vi "test Unpause timer reports the correct time.vi"(8 "error in (no error)":errorcluster, 11 "TestCase in":refnum<class "Test Unpause Timer.lvclass">) -> (0 "error out":errorcluster, 3 "TestCase out":refnum<class "Test Unpause Timer.lvclass">)   [LabVIEW 2018, in "Test Unpause Timer.lvclass"]
uses:
  Test Unpause Timer.lvclass
  Test Unpause Timer.lvclass/Test Unpause Timer.ctl
  <vilib>/addons/_JKI Toolkits/VI Tester/TestCase.llb/TestCase.lvclass
  C:/Program Files (x86)/National Instruments/LabVIEW 2018/vi.lib/addons/_JKI Toolkits/VI Tester/TestCase.llb/TestCase.lvclass
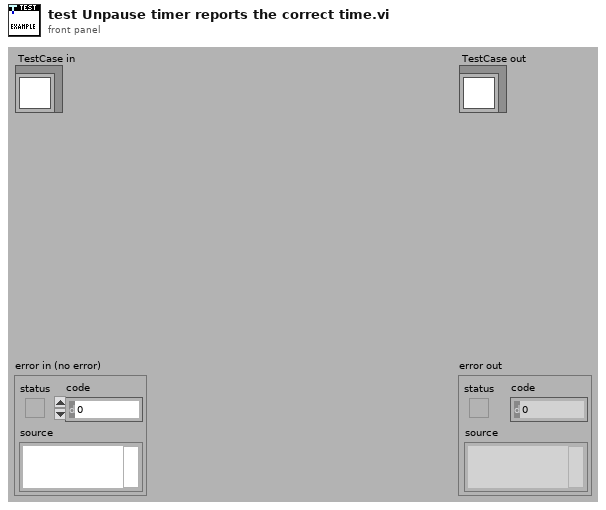
[diagram p1: front panel]
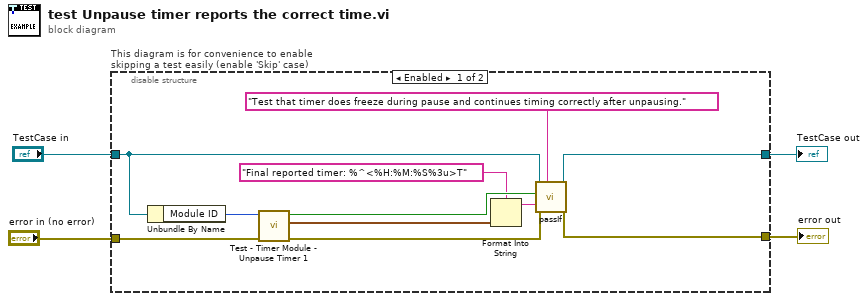
[diagram p0: block diagram]
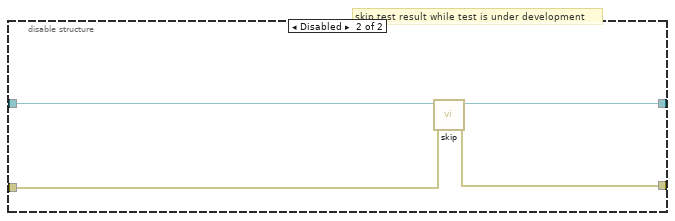
[diagram p2: hidden frame]
diagram:
  n1 = disable-structure "This diagram is for convenience to enable skipping a test easily (enable 'Skip' case)" shown="Enabled" {
    disable-tunnel: "TestCase in" -> [w11 w19]
    disable-tunnel: [w15 w17] -> w1
    disable-tunnel: [w14 w18] -> w3
    disable-tunnel: "error in (no error)" -> [w13 w16]
    frame Enabled {
      n2 = Unbundle By Name(w11) -> ("Module ID"=w10:i32)
      n3 = call "Test - Timer Module - Unpause Timer 1.vi"("error in (no error)"=w13, "Module ID"=w10) -> ("error out"=w12:errorcluster, "Final Timer"=w6:timestamp, "Pass"=w9:bool)  [unwired: 6 in, 1 out]
      n4 = Format Into String(format string="Final reported timer: %^<%H:%M:%S%3u>T", w6) -> (resulting string=w7:string)  [unwired: 2 in, 1 out]
      n5 = call-dynamic "passIf.vi"("custom report message (\"\")"="Test that timer does freeze during pause and continues timing correctly after unpausing." ("custom report message (\"\")"), "error in (no error)"=w12, "message (\"\")"=w7, "pass"=w9, "TestCase in"=w11) -> ("error out"=w14:errorcluster, "TestCase out"=w15:refnum<class "Test Unpause Timer.lvclass">)  [unwired: 5 in]
    }
    frame Disabled {
      # "skip test result while test is under development"
      n6 = call <vilib>:"skip.vi"("error in (no error)"=w16, "TestCase in"=w19) -> ("error out"=w18:errorcluster, "TestCase out"=w17:refnum<class "Test Unpause Timer.lvclass">)  [unwired: 8 in]
    }
  }
  "error out" <- w3
  "TestCase out" <- w1
